vi "JAI camera digital output including volet down.vi"(6 "AllSize":dbl, 8 "JAI camera fps":dbl, 10 "OG volAcquisitionTime":dbl, 11 "PFI 0 digital clock frequency":dbl) -> (1 "JAI camera digital output":bool[](array[boolean]))   [LabVIEW 2018]
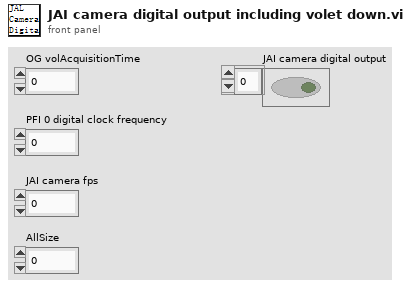
[diagram p1: front panel]
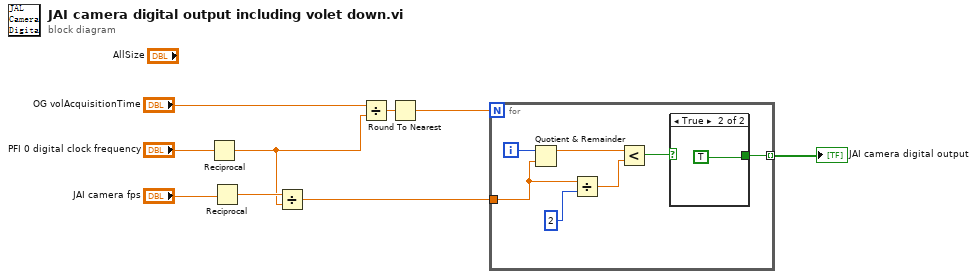
[diagram p0: block diagram]
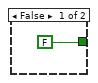
[diagram p2: hidden frame]
diagram:
  n1 = Reciprocal(x="PFI 0 digital clock frequency") -> (1/x=w3:dbl)
  n2 = Reciprocal(x="JAI camera fps") -> (1/x=w4:dbl)
  n3 = Divide(x=w4, y=w3) -> (x/y=w2:dbl)
  n4 = Divide(x="OG volAcquisitionTime", y=w3) -> (x/y=w5:dbl)
  n5 = Round To Nearest(number=w5) -> (nearest integer value=w1:dbl)
  n6 = for {
    N: w1 -> [_]
    tunnel: [w16] -> w9 mode=indexing
    tunnel: w2 -> [w12]
    i -> [w15]
    n7 = Quotient & Remainder(x=w15, y=w12) -> (x-y*floor(x/y)=w14:dbl)  [unwired: 1 out]
    n8 = Divide(x=w12, y=2) -> (x/y=w11:dbl)
    n9 = Less?(x=w14, y=w11) -> (x < y?=w10:bool)
    n10 = case shown="True" w10 {
      tunnel: [FALSE TRUE] -> w16
      frame False {
      }
      frame True {
      }
    }
  }
  "JAI camera digital output" <- w9
